vi "Move Tuner per VSWR.vi"(8 "error in (no error)":errorcluster, 9 "Timeout (s)":u8=60, 10 "VSWR and Phase":T1={"VSWR"=1.0, "Phase"=0.0}, 11 "iTuner reference in":refnum<k7>) -> (0 "error out":errorcluster, 2 "Current VSWR and Phase":dbl[][](array[numeric]), 3 "iTuner reference out":refnum<k7>)   [LabVIEW 2016, in "FocusTuner.lvlib"]
doc: "Adjusts the positions of the tuner axes to present the specified voltage standing wave ratio (VSWR) in magnitude and phase in the device reference plane with timeout."
uses:
  FocusTuner.lvlib
  Typedefs/VSWR and Phase.ctl
  <instrlib>/Focus iTuner Series/Public/Action-Status/Move Tuner per VSWR (VSWR and Phase).vi
  <instrlib>/Focus iTuner Series/Public/Data/Query VSWR (Current Position - All Frequencies).vi
  <instrlib>/Focus iTuner Series/Focus iTuner Series.lvlib
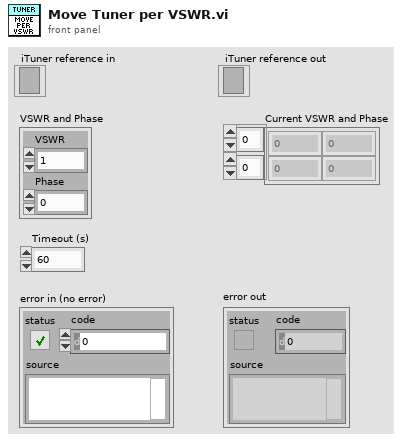
[diagram p1: front panel]
types:
  T1 = typedef "FocusTuner.lvlib/VSWR and Phase.ctl" = cluster{"VSWR":dbl, "Phase":dbl}
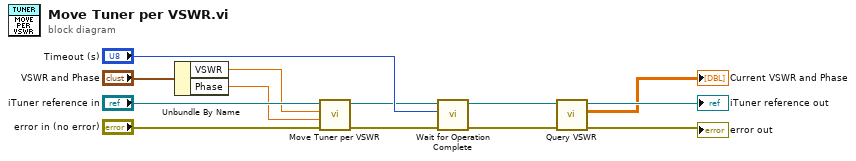
[diagram p0: block diagram]
diagram:
  n1 = Unbundle By Name("VSWR and Phase") -> ("VSWR"=w2:dbl, "Phase"=w1:dbl)
  n2 = call-poly <instrlib>:"Move Tuner per VSWR.vi"("error in (no error)"="error in (no error)", "Phase (0)"=w1, "VSWR (1)"=w2, "iTuner reference in"="iTuner reference in") -> ("error out"=w5:errorcluster, "iTuner reference out"=w6:refnum<k7>)  [unwired: 6 in]
  n3 = call <instrlib>:"Wait for Operation Complete.vi"("error in (no error)"=w5, "Timeout (60 s)"="Timeout (s)", "iTuner reference in"=w6) -> ("error out"=w3:errorcluster, "iTuner reference out"=w4:refnum<k7>)  [unwired: 7 in]
  n4 = call-poly <instrlib>:"Query VSWR.vi"("error in (no error)"=w3, "iTuner reference in"=w4) -> ("error out"=→"error out":errorcluster, "VSWR and Phase"=→"Current VSWR and Phase":dbl[][], "iTuner reference out"=→"iTuner reference out":refnum<k7>)  [unwired: 7 in]
